vi "Initialize.vi"(7 "Simulate":bool, 8 "error in (no error)":errorcluster, 9 "Reset (True)":bool=TRUE, 10 "ID Query (True)":bool=TRUE, 11 "VISA resource name":refnum<visa-resource-name>) -> (0 "error out":errorcluster, 3 "VISA resource name out":refnum<visa-resource-name>)   [LabVIEW 2018, in "Agilent U2722.lvlib"]
doc: "Establishes communication with the instrument and optionally performs an instrument identification query and/or an instrument reset. It also places the instrument in a default state needed for other instrument driver operations. Therefore, call this VI before calling other instrument driver VIs for this instrument. Generally, you need to call the Initialize VI only once at the beginning of an application."
uses:
  Agilent U2722.lvlib
panel:
  # "(c) 2009 National Instruments.  ALL RIGHTS RESERVED."
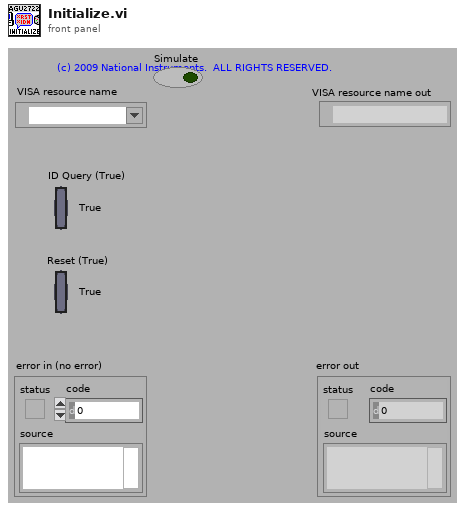
[diagram p1: front panel]
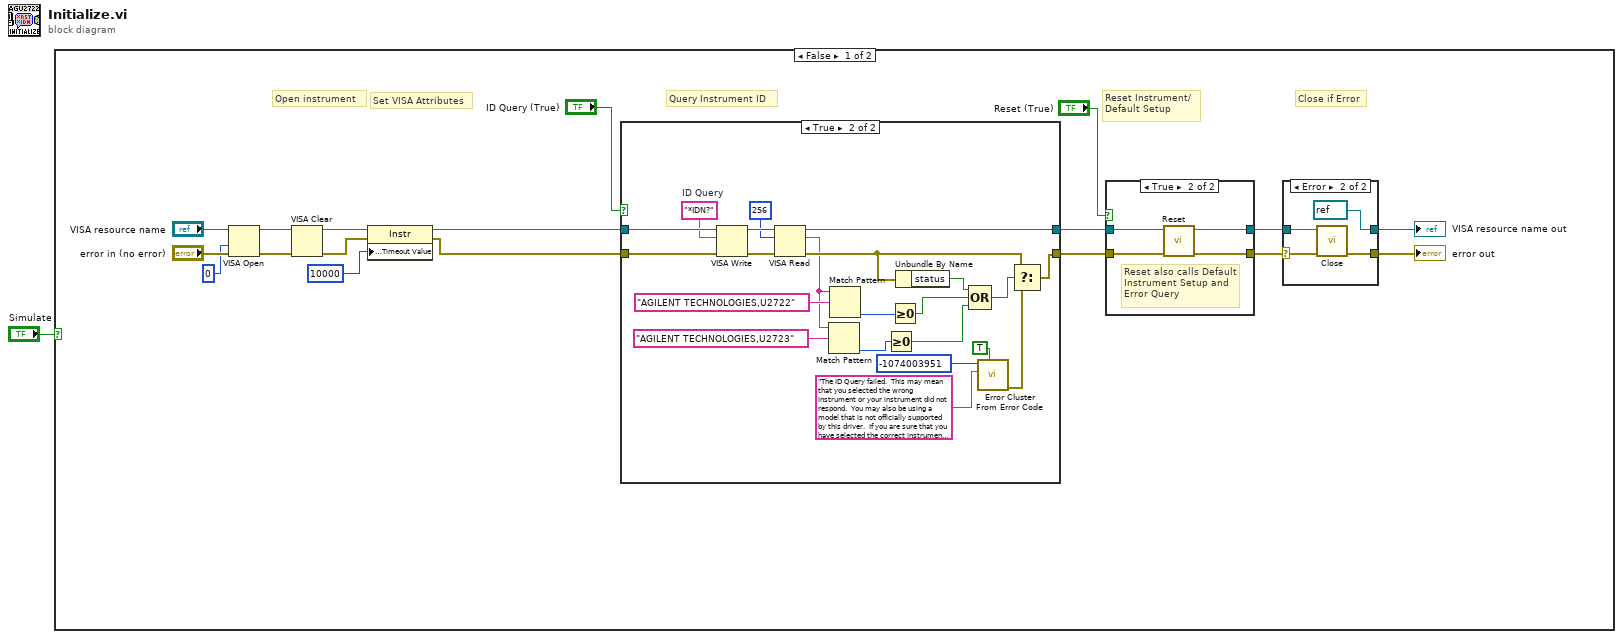
[diagram p0: block diagram]
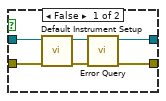
[diagram p3: hidden frame]
diagram:
  n1 = case shown="False" "Simulate" {
    frame False {
      # "Set VISA Attributes"
      # "Close if Error"
      # "Query Instrument ID"
      # "Reset Instrument/\nDefault Setup"
      # "Open instrument"
      n2 = VISA Open(access mode=u32 0, error in (no error)="error in (no error)", VISA resource name="VISA resource name") -> (VISA resource name=w11:refnum<visa-resource-name>, error out=w10:errorcluster)  [unwired: 2 in]
      n3 = VISA Clear(VISA resource name=w11, error in (no error)=w10) -> (VISA resource name out=w9:refnum<visa-resource-name>, error out=w8:errorcluster)
      n4 = property class="Instr"(reference=w9, error in=w8, "General Settings:Timeout Value"=u32 10000) -> (reference out=w3:refnum<visa-resource-name>, error out=w2:errorcluster)
      n5 = case shown="True" "ID Query (True)" {
        tunnel: [w36 w59] -> w18
        tunnel: [w37 w56] -> w19
        tunnel: w3 -> [w37 w57]
        tunnel: w2 -> [w36 w58]
        frame False {
        }
        frame True {
          w51 = "*IDN?"  # ID Query
          n6 = VISA Write(VISA resource name=w57, write buffer=w51, error in (no error)=w58) -> (VISA resource name out=w55:refnum<visa-resource-name>, error out=w54:errorcluster)  [unwired: 1 out]
          n7 = VISA Read(VISA resource name=w55, byte count=u32 256, error in (no error)=w54) -> (VISA resource name out=w56:refnum<visa-resource-name>, read buffer=w40:string, error out=w45:errorcluster)  [unwired: 1 out]
          n8 = Match Pattern(string=w40, regular expression="AGILENT TECHNOLOGIES,U2723") -> (offset past match=w39:i32)  [unwired: 1 in, 3 out]
          n9 = Match Pattern(string=w40, regular expression="AGILENT TECHNOLOGIES,U2722") -> (offset past match=w46:i32)  [unwired: 1 in, 3 out]
          n10 = Greater Or Equal To 0?(x=w39) -> (x >= 0?=w38:bool)
          n11 = Greater Or Equal To 0?(x=w46) -> (x >= 0?=w43:bool)
          n12 = Unbundle By Name(w45) -> ("status"=w44:bool)
          n13 = Compound Arithmetic op=OR(w44, w43, w38) -> (w42:bool)
          n14 = call <vilib>:"Error Cluster From Error Code.vi"("show call chain? (False)"=TRUE, "error message (\"\")"="The ID Query failed.  This may mean that you selected the wrong instrument or your instrument did not respond.  You may also be using a model that is not officially supported by this driver.  If you are sure that you have selected the correct instrument and it is responding, try disabling the ID Query." ("Source (VI Name)"), "error code (0)"=-1074003951 ("Code")) -> ("error out"=w50:errorcluster)  [unwired: 6 in]
          n15 = Select(t=w45, s=w42, f=w50) -> (s? t:f=w59:errorcluster)
        }
      }
      n16 = case shown="True" "Reset (True)" {
        tunnel: w18 -> [w30 w32]
        tunnel: [w27 w35] -> w4
        tunnel: w19 -> [w31 w33]
        tunnel: [w28 w34] -> w5
        frame False {
          n17 = call "Default Instrument Setup.vi"("error in (no error)"=w30, "VISA resource name"=w31) -> ("error out"=w26:errorcluster, "VISA resource name out"=w29:refnum<visa-resource-name>)  [unwired: 8 in]
          n18 = call "Error Query.vi"("error in (no error)"=w26, "VISA resource name"=w29) -> ("error out"=w27:errorcluster, "VISA resource name out"=w28:refnum<visa-resource-name>)  [unwired: 6 in, 2 out]
        }
        frame True {
          # "Reset also calls Default Instrument Setup and Error Query"
          n19 = call "Reset.vi"("error in (no error)"=w32, "VISA resource name"=w33) -> ("error out"=w35:errorcluster, "VISA resource name out"=w34:refnum<visa-resource-name>)  [unwired: 8 in]
        }
      }
      n20 = case shown="Error" w4 {
        selector: w4 -> [w20 w23]
        tunnel: w5 -> [w21 w24]
        tunnel: [w21 refnum<visa-resource-name> refnum ("VISA resource name out")] -> w7
        tunnel: [w20 w25] -> w6
        frame No Error {
        }
        frame Error {
          n21 = call "Close.vi"("error in (no error)"=w23, "VISA resource name"=w24) -> ("error out"=w25:errorcluster)  [unwired: 9 in]
        }
      }
      "VISA resource name out" <- w7
      "error out" <- w6
    }
    frame True {
    }
  }
